vi "FileSync.Update Sync.vi"(8 "error in (no error)":errorcluster, 9 "Sync Diff(F) or All(T)":bool caption="Sync Diff(F) or Force Copy All(T)", 10 "Normal(F)/Force Sync(T)":bool, 11 "File.Sync in":refnum<class "File.Sync.lvclass">) -> (0 "error out":errorcluster, 1 "Event Log":T2[](array[typedef]), 2 "Sync Items":T1[](array[typedef]), 3 "File.Sync out":refnum<class "File.Sync.lvclass">, 4 "Next Sync":dbl)   [LabVIEW 2024, in "EQMF.lvlib" / "File Utils.lvlib" / "File.Sync.lvclass"]
uses:
  File.Sync.lvclass
  File.Sync Item Log Record.ctl
  File.Sync Item Record.ctl
  File.Sync.lvclass/File.Sync.ctl
  File Utils.lvlib
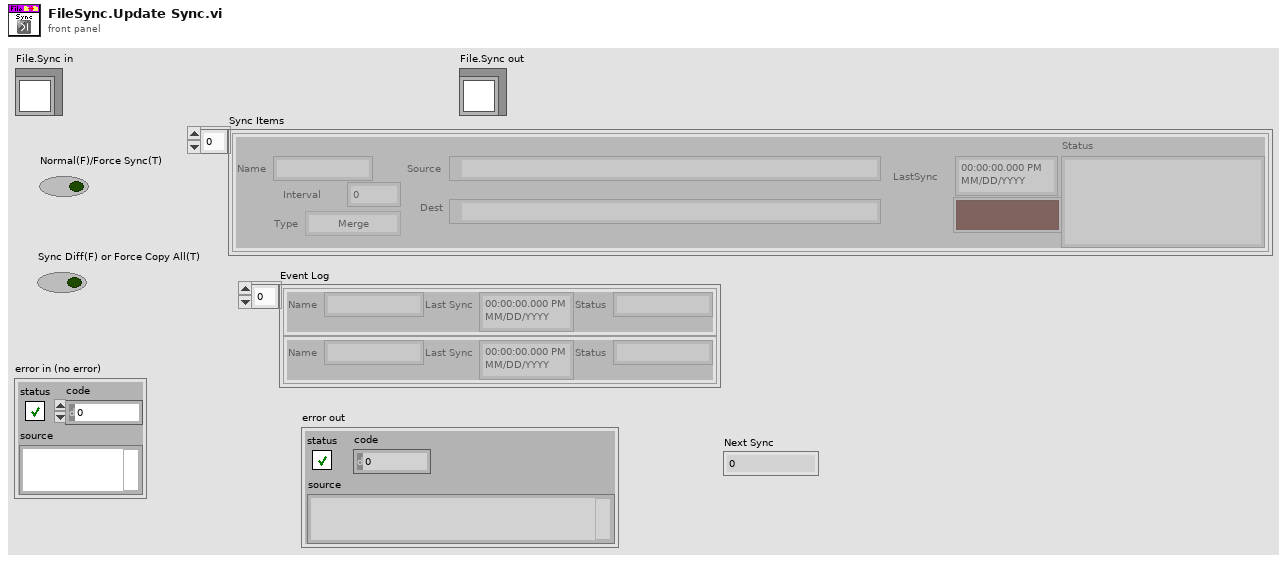
[diagram p1: front panel]
types:
  T1 = typedef "EQMF.lvlib/File Utils.lvlib/File.Sync.lvclass/File.Sync Item Record.ctl" = cluster{"Name":string, "Interval":dbl, "Source":path, "Dest":path, "LastSync":timestamp, "Status":string, "Error":bool, "Type":enum16{"Merge", "Match"}}
  T2 = typedef "EQMF.lvlib/File Utils.lvlib/File.Sync.lvclass/File.Sync Item Log Record.ctl" = cluster{"Name":string, "Last Sync":timestamp, "Status":string}
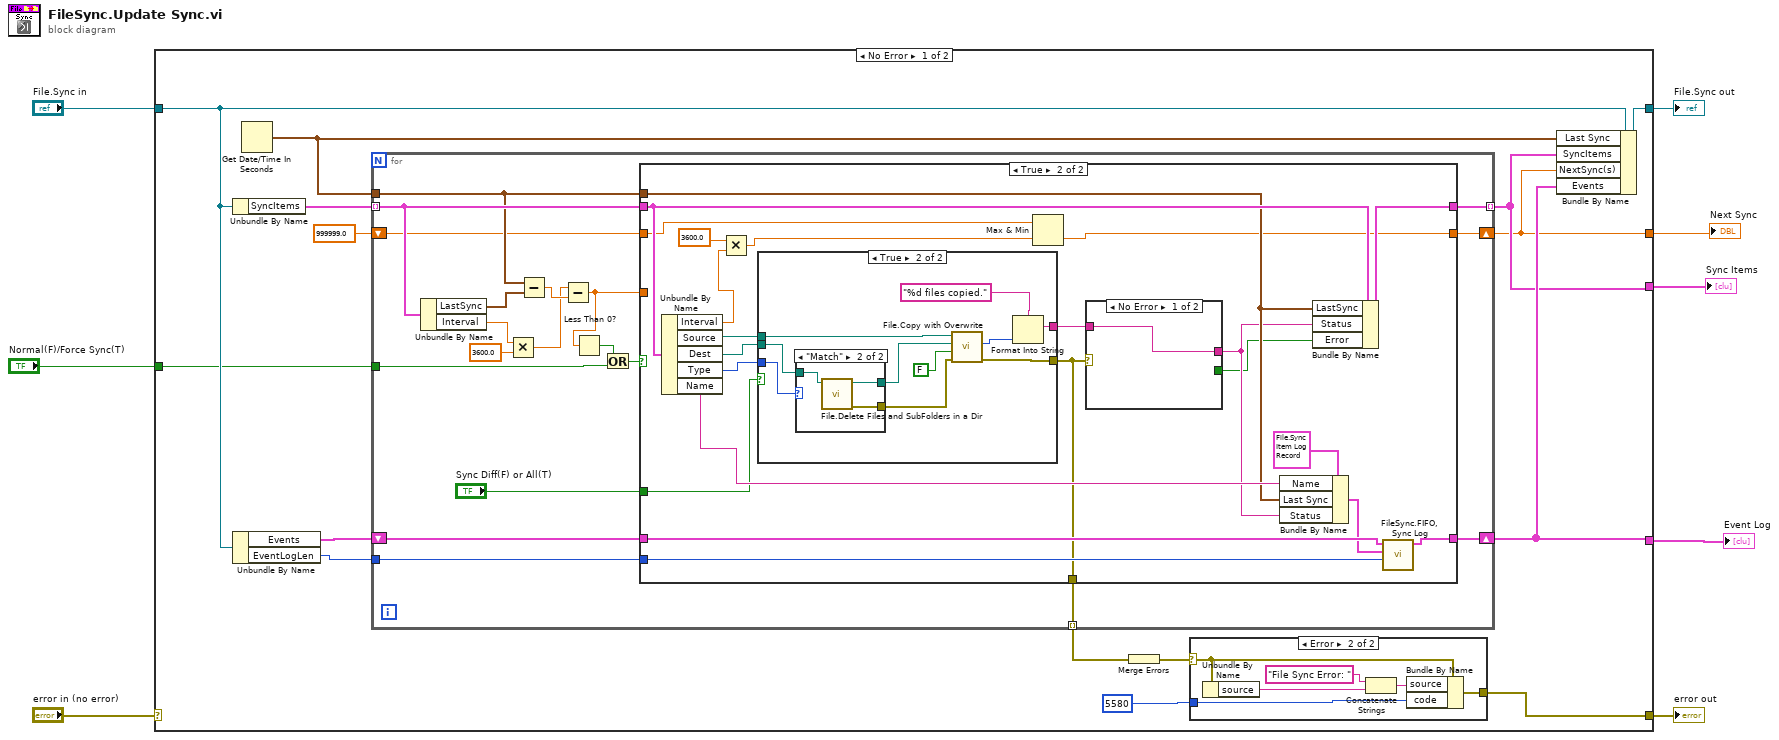
[diagram p0: block diagram]
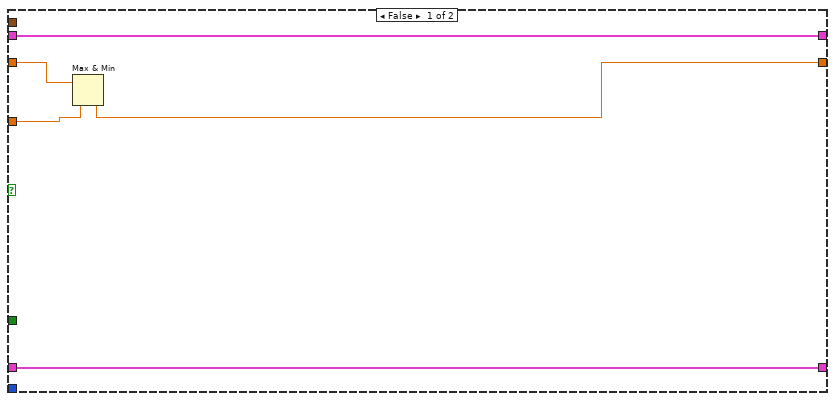
[diagram p3: hidden frame]
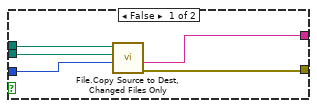
[diagram p4: hidden frame]
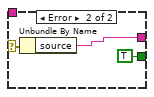
[diagram p6: hidden frame]
diagram:
  n1 = case shown="No Error" "error in (no error)" {
    selector: "error in (no error)" -> [_ w100]
    tunnel: [w9 w100] -> w7
    tunnel: [w23 w99] -> w5
    tunnel: "File.Sync in" -> [w20 w99]
    tunnel: "Normal(F)/Force Sync(T)" -> [w17 _]
    tunnel: [w15 _] -> w3
    tunnel: [w14 _] -> w2
    tunnel: [w13 _] -> w1
    frame No Error {
      n2 = Unbundle By Name(w20) -> ("SyncItems"=w22:T1[])
      n3 = Unbundle By Name(w20) -> ("Events"=w19:T2[], "EventLogLen"=w18:i32)
      n4 = Get Date/Time In Seconds() -> (seconds since 1Jan1904=w21:timestamp)
      n5 = for {
        tunnel: w22 -> [w47] mode=indexing
        tunnel: w21 -> [w43]
        shift-right: [w35] -> w15
        shift-left: w19 -> [w46]
        tunnel: w18 -> [w45]
        tunnel: [w44] -> w14 mode=indexing
        tunnel: w17 -> [w41]
        shift-right: [w36] -> w13
        shift-left: 999999.0 -> [w37]
        tunnel: [w34] -> w12 mode=indexing
        n6 = Unbundle By Name(w47) -> ("LastSync"=w48:timestamp, "Interval"=w32:dbl)
        n7 = Multiply(x=w32, y=3600.0) -> (x*y=w30:dbl)
        n8 = Subtract(x=w43, y=w48) -> (x-y=w39:dbl)
        n9 = Subtract(x=w30, y=w39) -> (x-y=w38:dbl)
        n10 = Less Than 0?(x=w38) -> (x < 0?=w40:bool)
        n11 = Or(x=w40, y=w41) -> (x .or. y?=w42:bool)
        n12 = case shown="True" w42 {
          tunnel: w47 -> [w52 w68]
          tunnel: w46 -> [w53 w73]
          tunnel: w45 -> [_ w72]
          tunnel: [w53 w71] -> w35
          tunnel: [w52 w67] -> w44
          tunnel: w43 -> [_ w65]
          tunnel: w38 -> [w50 _]
          tunnel: w37 -> [w51 w62]
          tunnel: [w49 w63] -> w36
          tunnel: [_ w61] -> w34
          tunnel: "Sync Diff(F) or All(T)" -> [_ w60]
          frame False {
            n13 = Max & Min(x=w51, y=w50) -> (min(x,y)=w49:dbl)  [unwired: 1 out]
          }
          frame True {
            n14 = Unbundle By Name(w68) -> ("Interval"=w55:dbl, "Source"=w75:path, "Dest"=w74:path, "Type"=w57:enum16{"Merge", "Match"}, "Name"=w69:string)
            n15 = Multiply(x=3600.0 ("y"), y=w55) -> (x*y=w54:dbl)
            n16 = case shown="True" w60 {
              tunnel: w75 -> [w80 w90]
              tunnel: w74 -> [w78 w83]
              tunnel: [w79 w89] -> w61
              tunnel: [w76 w85] -> w59
              tunnel: w57 -> [w77 w84]
              frame False {
                n17 = call "File.Copy Source to Dest, Changed Files Only.vi"("Type"=w77, "Dest Folder"=w78, "Source Folder"=w80) -> ("error out"=w79:errorcluster, "Report"=w76:string)  [unwired: 3 in, 4 out]
              }
              frame True {
                n18 = case shown="\"Match\"" w84 {
                  tunnel: w83 -> [w91 w94]
                  tunnel: [_ w93] -> w81
                  tunnel: [w91 w92] -> w82
                  frame "Merge", Default {
                  }
                  frame "Match" {
                    n19 = call "File.Delete Files and SubFolders in a Dir.vi"("Dir"=w94) -> ("error out"=w93:errorcluster, "Dup Dir"=w92:path)  [unwired: 9 in]
                  }
                }
                n20 = call "File.Copy with Overwrite.vi"("error in (no error)"=w81, "Dest is Dir(F)/File(T)"=FALSE, "Destination"=w82, "Source"=w90) -> ("error out"=w89:errorcluster, "Files Copied"=w86:i32)  [unwired: 5 in, 1 out]
                n21 = Format Into String(format string="%d files copied.", w86) -> (resulting string=w85:string)  [unwired: 2 in, 1 out]
              }
            }
            n22 = Max & Min(x=w62, y=w54) -> (min(x,y)=w63:dbl)  [unwired: 1 out]
            n23 = case shown="No Error" w61 {
              selector: w61 -> [_ w98]
              tunnel: [w95 w97] -> w64
              tunnel: w59 -> [w95 _]
              tunnel: [_ TRUE] -> w58
              frame No Error {
              }
              frame Error {
                n24 = Unbundle By Name(w98) -> ("source"=w97:string)
              }
            }
            n25 = Bundle By Name(cluster=T2 {"Name"="", "Last Sync"=timestamp(0 s since 1904-01-01), "Status"=""} ("New Event"), "Name"=w69, "Last Sync"=w65, "Status"=w64) -> (w66:T2)
            n26 = Bundle By Name(cluster=w68, "LastSync"=w65, "Status"=w64, "Error"=w58) -> (w67:T1)
            n27 = call "FileSync.FIFO, Sync Log.vi"("MaxLen"=w72, "New Event"=w66, "Array In"=w73) -> ("Array Out"=w71:T2[])  [unwired: 7 in, 1 out]
          }
        }
      }
      n28 = Merge Errors(w12) -> (w11:errorcluster)
      n29 = case shown="Error" w11 {
        selector: w11 -> [_ w26]
        tunnel: 5580 -> [_ w29]
        tunnel: [_ w24] -> w9
        frame No Error {
        }
        frame Error {
          n30 = Unbundle By Name(w26) -> ("source"=w25:string)
          n31 = Concatenate Strings("File Sync Error: ", w25) -> (w28:string)
          n32 = Bundle By Name(cluster=w26, "source"=w28, "code"=w29) -> (w24:errorcluster)
        }
      }
      n33 = Bundle By Name(cluster=w20, "Last Sync"=w21, "SyncItems"=w14, "NextSync(s)"=w13, "Events"=w15) -> (w23:refnum<class "File.Sync.lvclass">)
    }
    frame Error {
    }
  }
  "error out" <- w7
  "File.Sync out" <- w5
  "Event Log" <- w3
  "Sync Items" <- w2
  "Next Sync" <- w1
